vi "ConvertRudderCommand.vi"(1 "Rudder Command -5 to 5":dbl) -> (0 "Rudder Output Command":dbl)   [LabVIEW 2011]
uses:
  <vilib>/NXT/Dual Mode Library/prims/inRangeAndCoerce/inRangeAndCoerce_float.vi
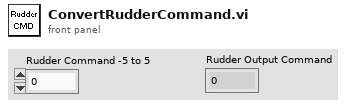
[diagram p1: front panel]
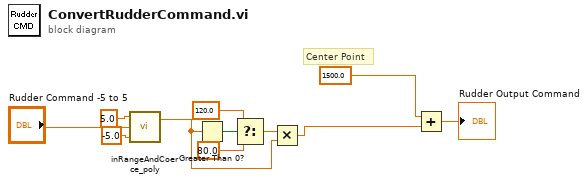
[diagram p0: block diagram]
diagram:
  # "Center Point"
  n1 = call-poly <vilib>:"inRangeAndCoerce_poly.vi"("lower limit"=-5.0, "x"="Rudder Command -5 to 5", "upper limit"=5.0) -> ("coerced(x)"=w2:dbl)  [unwired: 1 out]
  n2 = Greater Than 0?(x=w2) -> (x > 0?=w6:bool)
  n3 = Select(t=120.0, s=w6, f=80.0) -> (s? t:f=w3:dbl)
  n4 = Multiply(x=w3, y=w2) -> (x*y=w1:dbl)
  n5 = Add(x=1500.0 ("coerced(x)"), y=w1) -> (x+y=→"Rudder Output Command":dbl)
